vi "IHM_LaunchViByReference.vi"() -> (15 "error out":errorcluster)   [LabVIEW 2013]
doc: "This VI is the splash screen and launcher for the full-featured user interface. It performs the following operations:\n\n1. Opens reference to itself to pass to Full UI - Top-Level VI.vi. That VI will close the panel of this VI after it shows its own panel.\n2. Opens and runs runs Full UI - Top-Level VI.vi. This is done dynamically to improve the launch time of the application.\n3. Waits until Full UI - Top-Level VI.vi completes and closes the reference to that VI.\n4. If the VI is not running in a built application, reopens its panel.\n5. Closes the reference to itself.\n6. If the VI is running in a built application, exits the application."
panel:
  in  "ViToLaunch":refnum<vi>
  in  "error in (no error)":errorcluster caption="entrée d'erreur (pas d'erreur)"
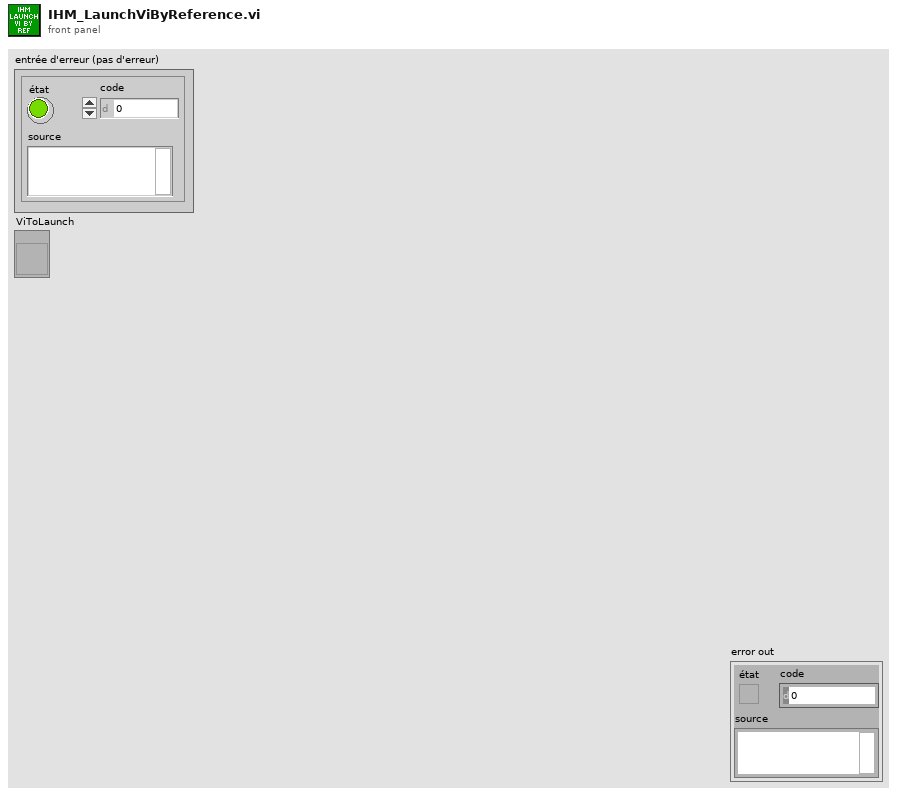
[diagram p1: front panel]
types:
  T1 = enum32{"invalid app kind", "Development System", "Run Time System", "Student Edition", "Embedded LabVIEW", "Evaluation", "Custom"}
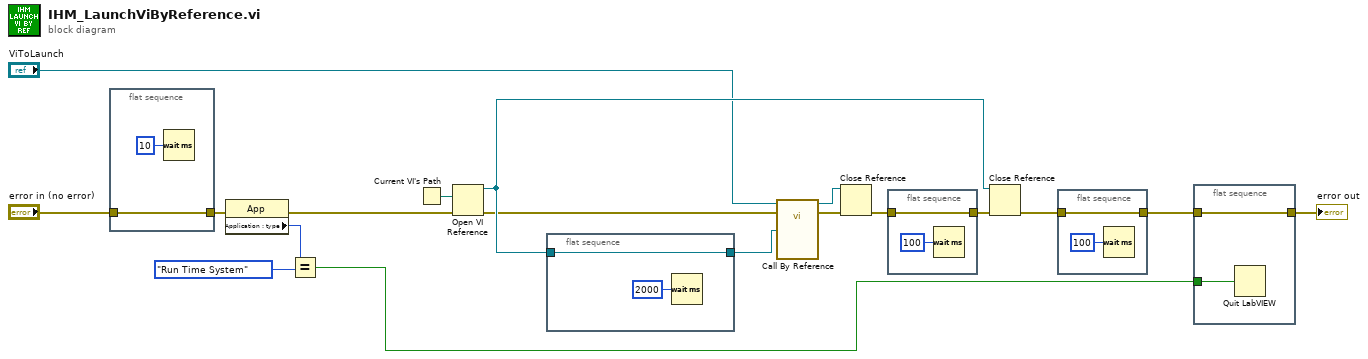
[diagram p0: block diagram]
diagram:
  n1 = flat-sequence {
    tunnel: [w20] -> w8
    tunnel: "error in (no error)" -> [w20]
    frame #0 {
      n2 = Wait (ms)(milliseconds to wait=u32 10 ("attente (ms)")) -> ()  [unwired: 1 out]
    }
  }
  n3 = property class="App"(error in=w8) -> (error out=w16:errorcluster, "Application : type"=w18:T1)  [unwired: 1 in, 1 out]
  n4 = Equal?(x=w18, y=T1."Run Time System") -> (x = y?=w9:bool)
  n5 = Current VI's Path() -> (path=w15:path)
  n6 = Open VI Reference(vi path=w15, error in (no error)=w16) -> (vi reference=w11:refnum<vi>, error out=w7:errorcluster)  [unwired: 1 in, 3 out]
  n7 = flat-sequence {
    tunnel: [w22] -> w12
    tunnel: w11 -> [w22]
    frame #0 {
      n8 = Wait (ms)(milliseconds to wait=u32 2000 ("attente (ms)")) -> ()  [unwired: 1 out]
    }
  }
  n9 = call-by-ref "?"(reference="ViToLaunch", error in=w7, "LauncherRef"=w12) -> (reference out=w13:refnum<vi>, error out=w14:errorcluster)  [unwired: 10 in, 1 out]
  n10 = Close Reference(reference=w13, error in (no error)=w14) -> (error out=w5:errorcluster)
  n11 = flat-sequence {
    tunnel: [w24] -> w6
    tunnel: w5 -> [w24]
    frame #0 {
      n12 = Wait (ms)(milliseconds to wait=u32 100 ("attente (ms)")) -> ()  [unwired: 1 out]
    }
  }
  n13 = Close Reference(reference=w11, error in (no error)=w6) -> (error out=w4:errorcluster)
  n14 = flat-sequence {
    tunnel: [w26] -> w3
    tunnel: w4 -> [w26]
    frame #0 {
      n15 = Wait (ms)(milliseconds to wait=u32 100 ("attente (ms)")) -> ()  [unwired: 1 out]
    }
  }
  n16 = flat-sequence {
    tunnel: [w28] -> w10
    tunnel: w3 -> [w28]
    tunnel: w9 -> [w27]
    frame #0 {
      n17 = Quit LabVIEW(quit? (T)=w27) -> ()
    }
  }
  "error out" <- w10
